vi "HEWH Variable Purge Temps.vi"(6 "Disable Purge Pressurization":bool, 9 "State":T1, 10 "GPM Target":T2 format="%.2f", 11 "Temperature Input (F)":T2 format="%.2f") -> (3 "Temperature Output (F)":T2 format="%.2f")   [LabVIEW 2020]
uses:
  Utility/Custom Pallet Controls/Custom Pallet DBL.ctl
  Type Definitions/HEWH Purge Draw.ctl
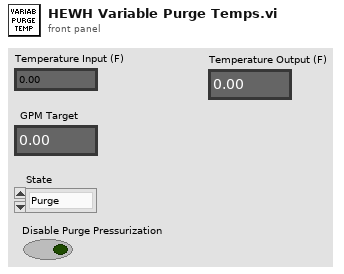
[diagram p1: front panel]
types:
  T1 = typedef "HEWH Purge Draw.ctl" = enum16{"Purge", "Draw"}
  T2 = typedef "Custom Pallet DBL.ctl" = dbl
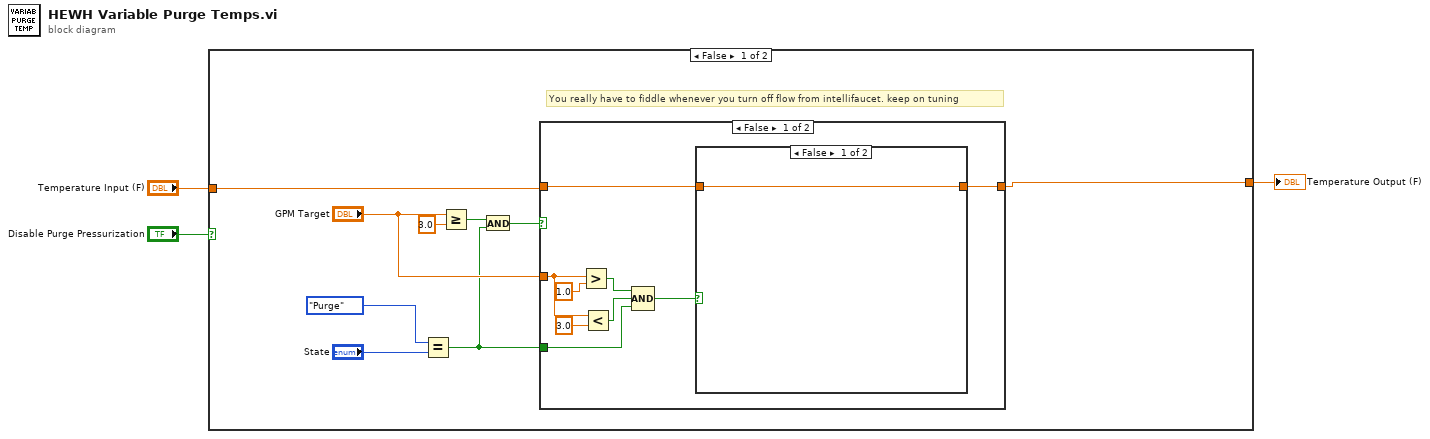
[diagram p0: block diagram]
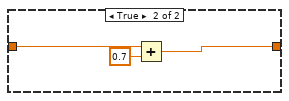
[diagram p2: hidden frame]
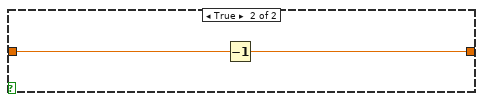
[diagram p3: hidden frame]
diagram:
  n1 = case shown="False" "Disable Purge Pressurization" {
    tunnel: [w5 w28] -> w3
    tunnel: "Temperature Input (F)" -> [w4 w28]
    frame False {
      # "You really have to fiddle whenever you turn off flow from intellifaucet. keep on tuning"
      n2 = Equal?(x=HEWH_Purge_Draw."Purge", y="State") -> (x = y?=w6:bool)
      n3 = Greater Or Equal?(x="GPM Target", y=3.0) -> (x >= y?=w8:bool)
      n4 = And(x=w8, y=w6) -> (x .and. y?=w9:bool)
      n5 = case shown="False" w9 {
        tunnel: w4 -> [w14 w27]
        tunnel: [w13 w26] -> w5
        tunnel: "GPM Target" -> [w20 _]
        tunnel: w6 -> [w16 _]
        frame False {
          n6 = Greater?(x=w20, y=1.0) -> (0:w18:bool)
          n7 = Less?(x=w20, y=3.0) -> (x < y?=w17:bool)
          n8 = Compound Arithmetic op=AND(w18, w17, w16) -> (w15:bool)
          n9 = case shown="False" w15 {
            tunnel: w14 -> [w22 w25]
            tunnel: [w22 w23] -> w13
            frame False {
            }
            frame True {
              n10 = Add(x=w25, y=0.7) -> (x+y=w23:T2)
            }
          }
        }
        frame True {
          n11 = Decrement(x=w27) -> (x-1=w26:T2)
        }
      }
    }
    frame True {
    }
  }
  "Temperature Output (F)" <- w3
